vi "Read configuration.vi"(8 "error in":errorcluster, 11 "ExampleStateMachine editor node in":refnum<class "ExampleStateMachine editor node.lvclass">) -> (0 "error out":errorcluster, 2 "configuration":refnum<class "NISE_CEF_serializable configuration.lvclass">, 3 "ExampleStateMachine editor node out":refnum<class "ExampleStateMachine editor node.lvclass">)   [LabVIEW 2017, in "ExampleStateMachine editor node.lvclass"]
uses:
  ExampleStateMachine editor node.lvclass
  <vilib>/NI/Configuration Framework/serializable configuration/NISE_CEF_serializable configuration.lvclass
  ExampleStateMachine editor node.lvclass/ExampleStateMachine editor node.ctl
  module/configuration/ExampleStateMachine configuration.lvclass
  C:/Program Files (x86)/National Instruments/LabVIEW 2017/vi.lib/NI/Configuration Framework/serializable configuration/NISE_CEF_serializable configuration.lvclass
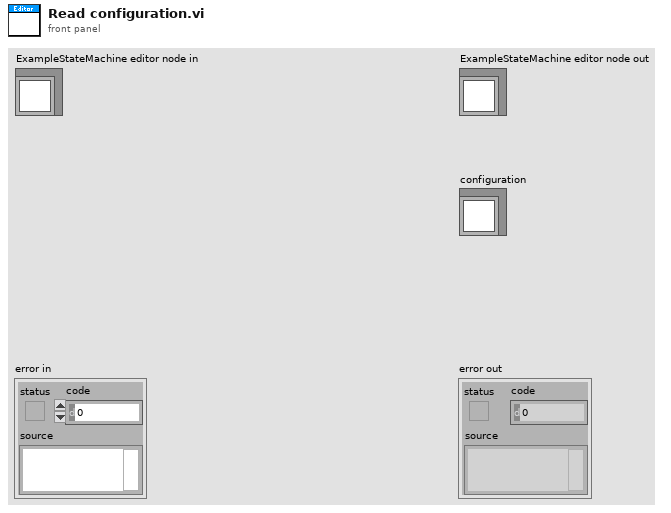
[diagram p1: front panel]
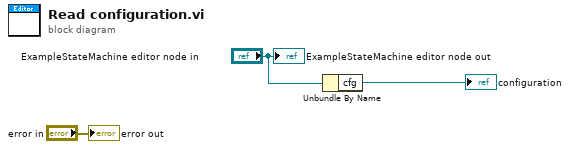
[diagram p0: block diagram]
diagram:
  n1 = Unbundle By Name("ExampleStateMachine editor node in") -> ("cfg"=→"configuration":refnum<class "ExampleStateMachine configuration.lvclass">)
  "error out" <- "error in"
  "ExampleStateMachine editor node out" <- "ExampleStateMachine editor node in"
